vi "EmptyPlugin_Interface.vi"(9 "EventsIn":T1, 10 "Events":T2) -> ()   [LabVIEW 2014, in "_EmptyPlugin.lvclass"]
uses:
  _EmptyPlugin.lvclass
  _LVCMPlugin/GCMPlugin_EventsOut.ctl
  _LVCMPlugin/GCMPlugin_EventsIn.ctl
  GCMPlugin/GCMPlugin.lvclass
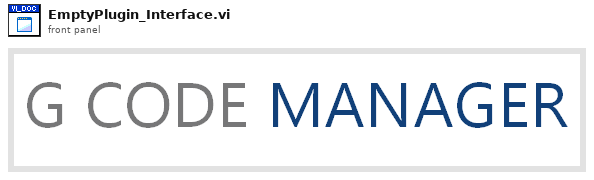
[diagram p1: front panel]
types:
  T1 = typedef "GCMPlugin.lvclass/GCMPlugin_EventsIn.ctl" = cluster{"Stop":refnum<user-event>, "ItemSelected":refnum<user-event>, "ItemDeselected":refnum<user-event>, "PluginActivated":refnum<user-event>, "PluginDeactivated":refnum<user-event>}
  T2 = typedef "GCMPlugin.lvclass/GCMPlugin_EventsOut.ctl" = cluster{"ItemEdited":refnum<user-event>}
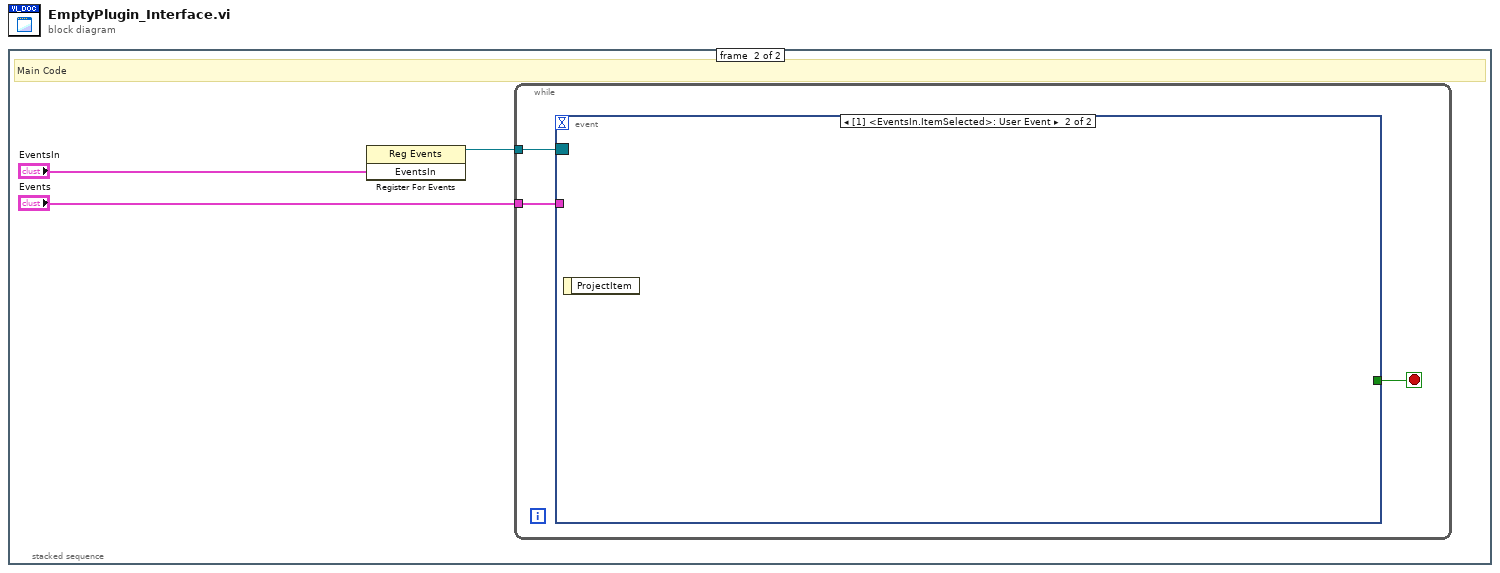
[diagram p0: block diagram]
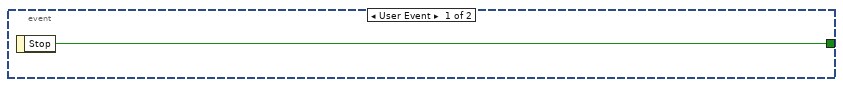
[diagram p3: hidden frame]
diagram:
  n1 = stacked-sequence {
    frame #0 {
      # "Init"
    }
    frame #1 {
      # "Main Code"
      n2 = register-events("EventsIn") -> (reference out=w2:refnum<event-registration>)  [unwired: 2 in, 1 out]
      n3 = while {
        tunnel: w2 -> [w6]
        tunnel: "Events" -> [w5]
        stop <- w4 stop-if-true
        n4 = event shown="[1] <EventsIn.ItemSelected>: User Event" {
          selector: w6 -> [_ _]
          dyn-events: _ -> [_ _]
          timeout: _ -> [_ _]
          tunnel: w5 -> [_ _]
          tunnel: [w7 _] -> w4
          event User Event {
            n5 = event-data() -> ("Stop"=w7:bool)  [unwired: 1 in]
          }
          event User Event {
            n6 = event-data() -> ()  [unwired: 1 in, 1 out]
          }
        }
      }
    }
  }
